vi "Run Stop Module.vi"(8 "error in":errorcluster, 10 "Module ID":i32=-1, 11 "Event vi Ref":refnum<vi>) -> (0 "error out":errorcluster)   [LabVIEW 2020, in "DQMH_API.lvlib"]
doc: "This VI checks the Main.vi State of the selected DQMH Module"
uses:
  DQMH_API.lvlib
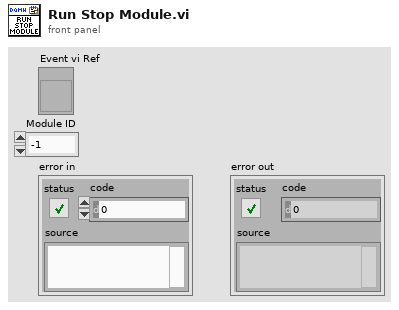
[diagram p1: front panel]
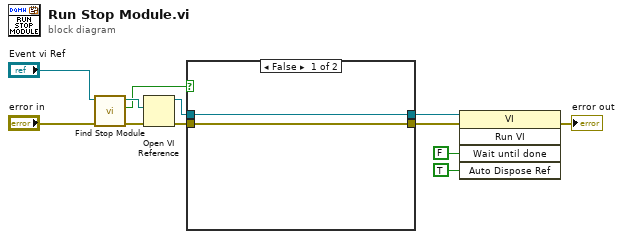
[diagram p0: block diagram]
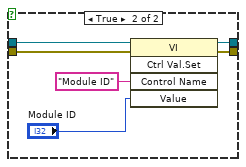
[diagram p2: hidden frame]
diagram:
  n1 = call "Find Stop Module.vi"("error in"="error in", "Event vi Ref"="Event vi Ref") -> ("error out"=w10:errorcluster, "Cloneable?"=w1:bool, "Stop Module"=w7:path)  [unwired: 7 in]
  n2 = Open VI Reference(vi path=w7, error in (no error)=w10) -> (vi reference=w5:refnum<vi>, error out=w3:errorcluster)  [unwired: 4 in]
  n3 = case shown="False" w1 {
    tunnel: w5 -> [w14 w20]
    tunnel: [w14 w19] -> w4
    tunnel: w3 -> [w13 w18]
    tunnel: [w13 w17] -> w2
    frame False {
    }
    frame True {
      n4 = invoke class="VI" method="Ctrl Val.Set"(reference=w20, error in=w18, "Control Name"="Module ID", "Value"="Module ID") -> (reference out=w19:refnum<vi>, error out=w17:errorcluster)  [unwired: 1 in, 3 out]
    }
  }
  n5 = invoke class="VI" method="Run VI"(reference=w4, error in=w2, "Wait until done"=FALSE ("Wait Until Done"), "Auto Dispose Ref"=TRUE ("Auto Dispose Reference")) -> (error out=→"error out":errorcluster)  [unwired: 1 in, 4 out]
